vi "readRegisterS0_32.vi"(8 "error in (no error)":errorcluster, 10 "Offset":u32) -> (0 "error out":errorcluster, 3 "Data 1":u32=255)   [LabVIEW 2015, in "ESLSCDLL.lvlib"]
uses:
  ESLSCDLL.lvlib
  Globals.vi
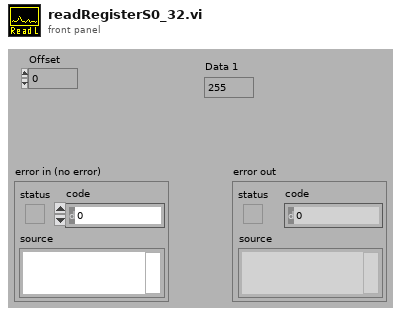
[diagram p1: front panel]
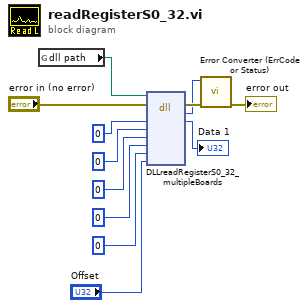
[diagram p0: block diagram]
diagram:
  n1 = global read "Globals.vi" "dll path"() -> (w1:path)
  n2 = dll-call lib="C:/ENTW/PCIE/LV64/board.vis/ESLSCDLL.dll" fn="DLLreadRegisterS0_32_multipleBoards" ("lwlscdll.dll:DLLReadLongS0")(path in=w1, error in="error in (no error)", "data0"=u32 0 ("data"), "data1"=u32 0, "data2"=u32 0, "data3"=u32 0, "data4"=u32 0, "address"="Offset") -> (error out=w8:errorcluster, "es_status_codes"=w7:i32, "data0"=→"Data 1":u32)  [unwired: 6 in, 1 out]
  n3 = call "Error Converter (ErrCode or Status).vi"("error in (no error)"=w8, "error code"=w7) -> ("error out"=→"error out":errorcluster)  [unwired: 9 in]
